vi "GetBuiltPath.vi"(3 "Standard Output":string) -> (1 "Built Path":path)   [LabVIEW 2020, in "Package Builder.lvlib"]
uses:
  Package Builder.lvlib
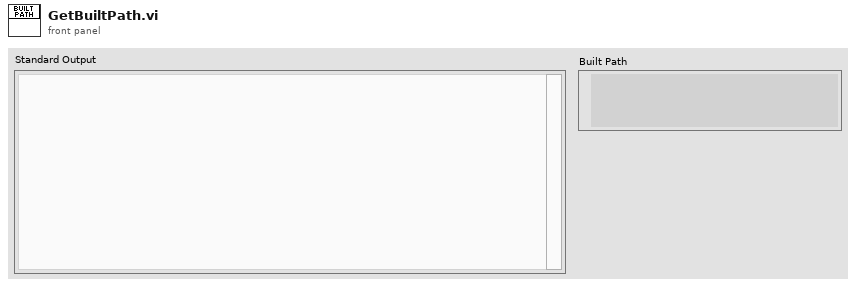
[diagram p1: front panel]
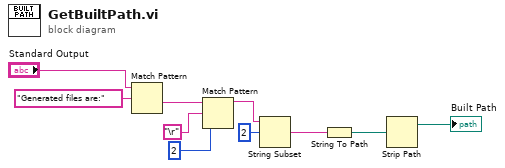
[diagram p0: block diagram]
diagram:
  n1 = Match Pattern(string="Standard Output", regular expression="Generated files are:") -> (after substring=w8:string)  [unwired: 1 in, 3 out]
  n2 = Match Pattern(string=w8, regular expression="\r", offset (0)=2) -> (before substring=w5:string)  [unwired: 3 out]
  n3 = String Subset(string=w5, offset (0)=2) -> (substring=w3:string)  [unwired: 1 in]
  n4 = String To Path(string=w3) -> (path=w2:path)
  n5 = Strip Path(path=w2) -> (stripped path=→"Built Path":path)  [unwired: 1 out]
